vi "Panel Event.vi"(10 "Events":T1, 11 "SubProcess in":refnum<class "SubProcess.lvclass">) -> (0 "error out":errorcluster, 3 "SubProcess out":refnum<class "SubProcess.lvclass">)   [LabVIEW 2021, in "SubProcess.lvlib" / "SubProcess.lvclass"]
uses:
  SubProcess.lvclass
  Panel Event/Events.ctl
  SubProcess.lvclass/SubProcess.ctl
  Panel Event/Panel Event.lvlib
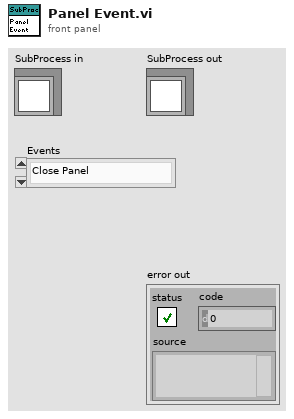
[diagram p1: front panel]
types:
  T1 = typedef "Panel Event.lvlib/Events.ctl" = enum16{"Close Panel", "Show Panel", "Hide Panel"}
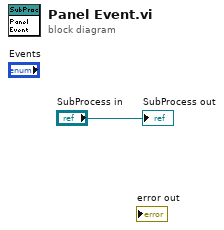
[diagram p0: block diagram]
diagram:
  "SubProcess out" <- "SubProcess in"
